vi "Ventilador.vi"() -> ()   [LabVIEW 2020]
panel:
  out "Ventilador":bool
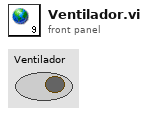
[diagram p1: front panel]
diagram:
